vi "Login Success.vi"(8 "error in (no error)":errorcluster, 10 "username":string, 11 "[Data] Userinfo Binary in":refnum<class "[Data] Userinfo Binary.lvclass">) -> (0 "error out":errorcluster, 3 "[Data] Userinfo Binary out":refnum<class "[Data] Userinfo Binary.lvclass">)   [LabVIEW 2020, in "[Data] Userinfo Binary.lvclass"]
uses:
  [Data] Userinfo Binary.lvclass
  [Data] Userinfo Binary.lvclass/[Data] Userinfo Binary.ctl
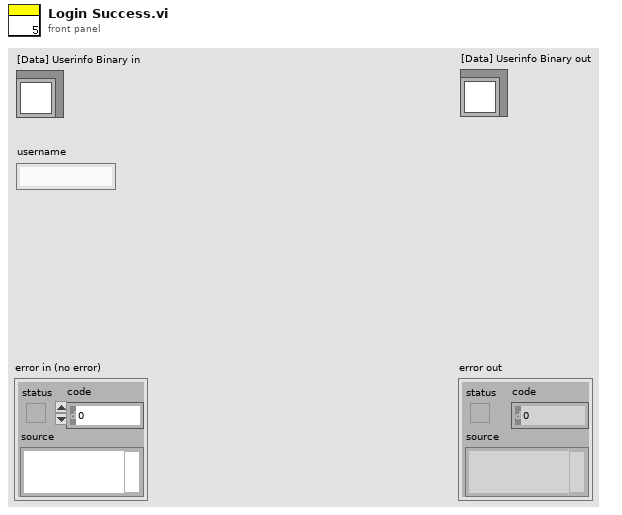
[diagram p1: front panel]
types:
  T1 = typedef "[Data] Userinfo Binary.lvclass/user info.ctl" = cluster{"password":string, "authority":i8, "department":string, "post":string, "remark":string, "create time":timestamp, "last login time":timestamp}
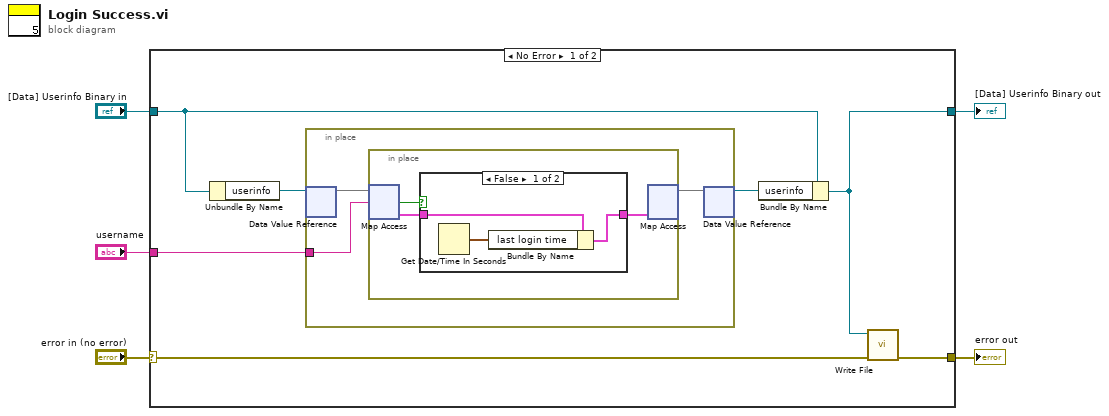
[diagram p0: block diagram]
diagram:
  n1 = case shown="No Error" "error in (no error)" {
    selector: "error in (no error)" -> [w10 w24]
    tunnel: [w9 w24] -> w2
    tunnel: "[Data] Userinfo Binary in" -> [w11 w23]
    tunnel: [w8 w23] -> w4
    tunnel: "username" -> [w12 _]
    frame No Error {
      n2 = Unbundle By Name(w11) -> ("userinfo"=w7:refnum<data-value>)
      n3 = in-place {
        in-place-border: w12 -> [w15]
        n4 = in-place-dvr #1(w7) -> (w14:map{string, T1})  [unwired: 1 out]
        n5 = in-place {
          n6 = in-place-map #2(w14, w15) -> (w18:T1, w17:bool)  [unwired: 1 in]
          n7 = case shown="False" w17 {
            tunnel: w18 -> [w21 w22]
            tunnel: [w20 w22] -> w16
            frame False {
              n8 = Get Date/Time In Seconds() -> (seconds since 1Jan1904=w19:timestamp)
              n9 = Bundle By Name(cluster=w21, "last login time"=w19) -> (w20:T1)
            }
            frame True {
            }
          }
          n10 = in-place-map #2(w16) -> (w13:map{string, T1})  [unwired: 1 in, 2 out]
        }
        n11 = in-place-dvr #1(w13) -> (w6:refnum<data-value>)  [unwired: 1 out]
      }
      n12 = Bundle By Name(cluster=w11, "userinfo"=w6) -> (w8:refnum<class "[Data] Userinfo Binary.lvclass">)
      n13 = call "Write File.vi"("error in (no error)"=w10, "[Data] Userinfo Binary in"=w8) -> ("error out"=w9:errorcluster)  [unwired: 8 in, 1 out]
    }
    frame Error {
    }
  }
  "error out" <- w2
  "[Data] Userinfo Binary out" <- w4
